vi "HXG2daqFGV.vi"(7 "daqFGV":T2, 8 "error in (no error)":errorcluster) -> (0 "error out":errorcluster, 3 "MAX":T1)   [LabVIEW 2012]
uses:
  HXG2daq.ctl
  Controls/HXG2_MaxConstants.ctl
  <vilib>/DAQmx/write.llb/DAQmx Write (Digital 1D Bool NChan 1Samp 1Line).vi
  <vilib>/DAQmx/write.llb/DAQmx Write (Analog 1D DBL NChan 1Samp).vi
  <resource>/objmgr/daqmx.rc
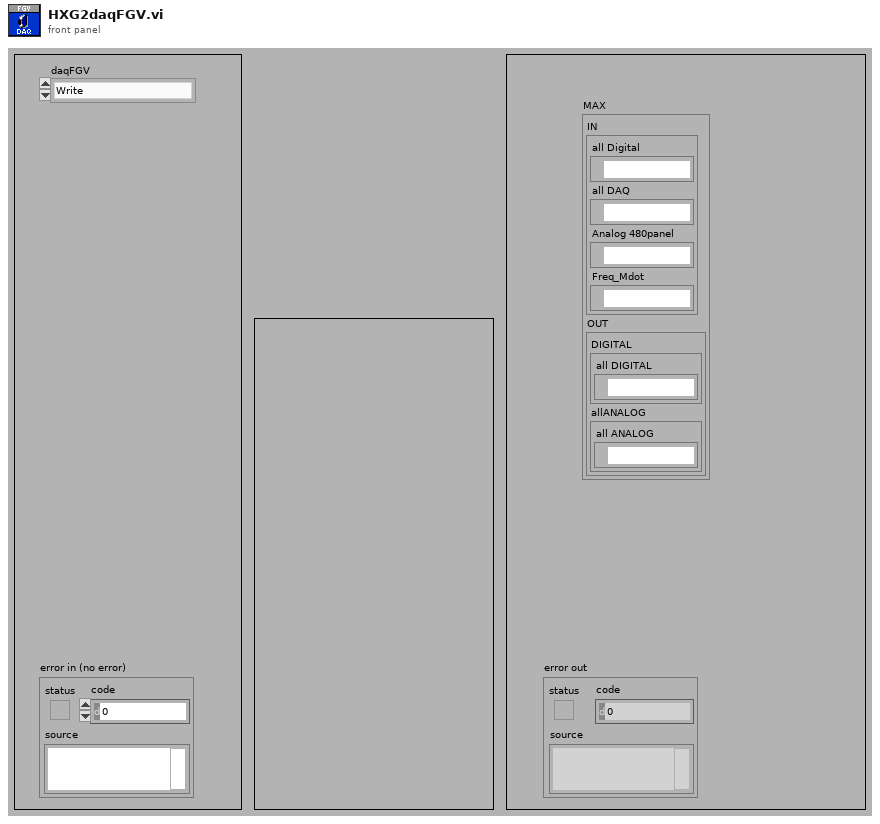
[diagram p1: front panel]
types:
  T1 = typedef "HXG2_MaxConstants.ctl" = cluster{"IN":cluster{"all Digital":refnum<k21>, "all DAQ":refnum<k21>, "Analog 480panel":refnum<k21>, "Freq_Mdot":refnum<k21>}, "OUT":cluster{"DIGITAL":cluster{"all DIGITAL":refnum<k21>}, "allANALOG":cluster{"all ANALOG":refnum<k21>}}}
  T2 = typedef "HXG2daq.ctl" = enum16{"Write", "Pass", "Initialize", "Stop"}
  T3 = cluster{"all Digital":refnum<k21>, "all DAQ":refnum<k21>, "Analog 480panel":refnum<k21>, "Freq_Mdot":refnum<k21>}
  T4 = cluster{"[0]":refnum<k21>, "[1]":refnum<k21>, "[2]":refnum<k21>, "[3]":refnum<k21>}
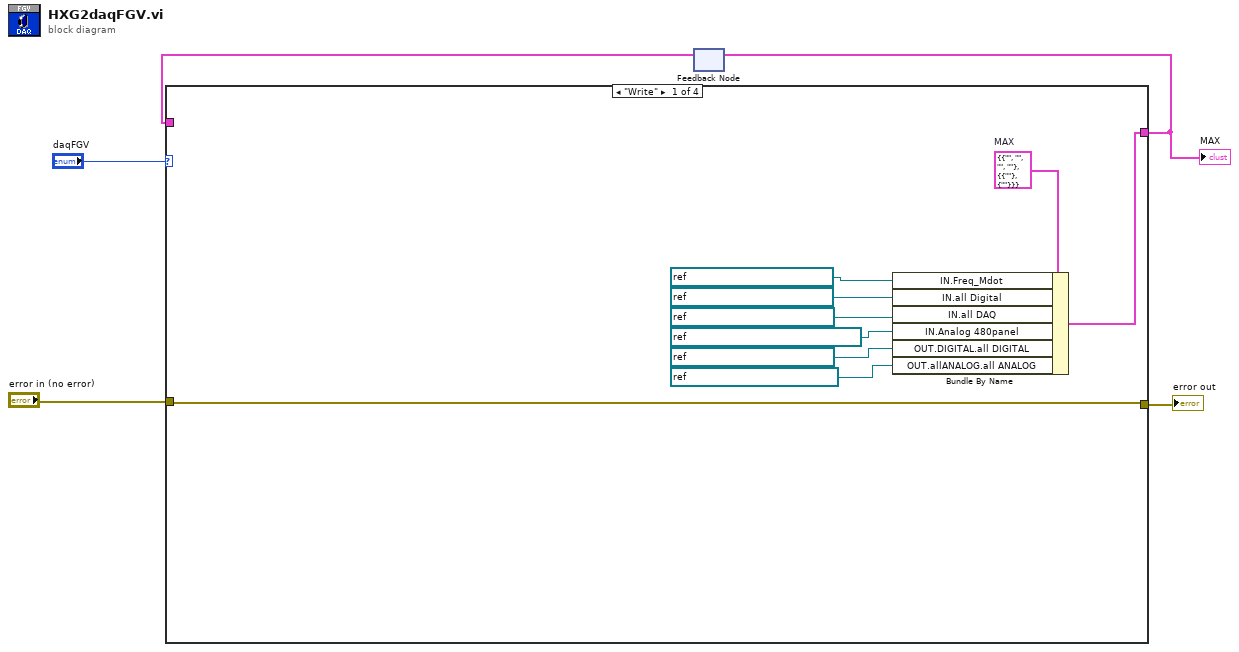
[diagram p0: block diagram]
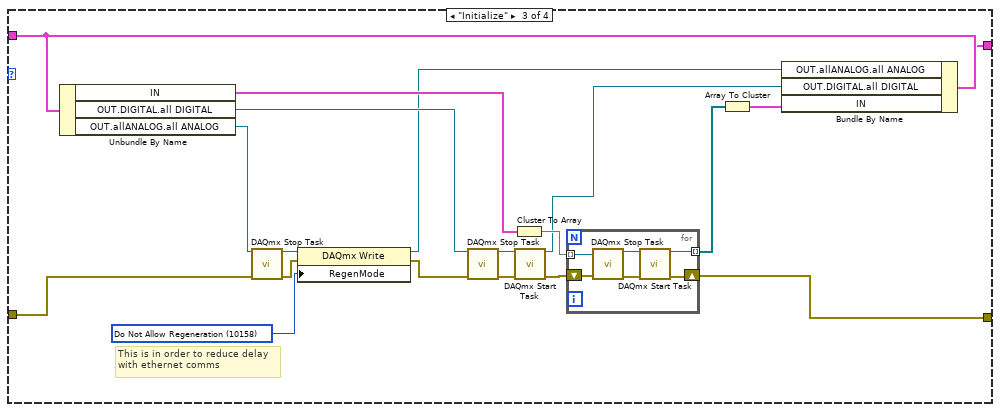
[diagram p3: hidden frame]
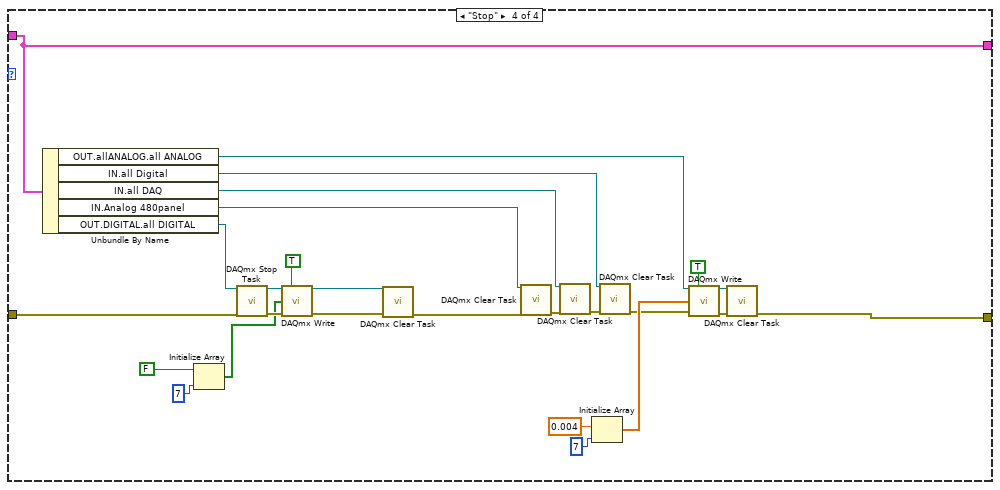
[diagram p4: hidden frame]
diagram:
  n1 = feedback #1() -> (w2:T1)  [unwired: 1 in]
  n2 = case shown="\"Write\"" "daqFGV" {
    tunnel: "error in (no error)" -> [w14 w15 w22 w62]
    tunnel: [w14 w15 w31 w53] -> w4
    tunnel: [w9 w16 w28 w67] -> w3
    tunnel: w2 -> [_ w16 w29 w67]
    frame "Write" {
      w13 = T1 {"IN"={"all Digital"="", "all DAQ"="", "Analog 480panel"="", "Freq_Mdot"=""}, "OUT"={"DIGITAL"={"all DIGITAL"=""}, "allANALOG"={"all ANALOG"=""}}}  # MAX
      n3 = Bundle By Name(cluster=w13, "IN.Freq_Mdot"=refnum<k21> "HX_Cal2_FeqMdot" ("all Digital"), "IN.all Digital"=refnum<k21> "HXCal1_IN_allDIGITAL" ("all Digital"), "IN.all DAQ"=refnum<k21> "HXCal2_IN_ANALOG" ("all DAQ"), "IN.Analog 480panel"=refnum<k21> "HXCal1_IN_ANALOG_480Panel" ("all TC"), "OUT.DIGITAL.all DIGITAL"=refnum<k21> "HXCal1_OUT_allDIGITAL" ("all DIGITAL"), "OUT.allANALOG.all ANALOG"=refnum<k21> "HX_Cal1_OUT_allANALOG" ("all ANALOG")) -> (w9:T1)
    }
    frame "Pass" {
    }
    frame "Initialize" {
      w17 = 10158 items=["Allow Regeneration"=10097, "Do Not Allow Regeneration"=10158] ("RegenMode")
      # "This is in order to reduce delay\nwith ethernet comms"
      n4 = Unbundle By Name(w29) -> ("IN"=w34:T3, "OUT.DIGITAL.all DIGITAL"=w30:refnum<k21>, "OUT.allANALOG.all ANALOG"=w32:refnum<k21>)
      n5 = call <vilib>:"DAQmx Stop Task.vi"("task/channels in"=w32, "error in"=w22) -> ("task out"=w20:refnum<k21>, "error out"=w21:errorcluster)  [unwired: 12 in]
      n6 = property class="DAQmx Write"(reference=w20, error in=w21, "RegenMode"=w17) -> (reference out=w18:refnum<k21>, error out=w19:errorcluster)
      n7 = call <vilib>:"DAQmx Stop Task.vi"("task/channels in"=w30, "error in"=w19) -> ("task out"=w24:refnum<k21>, "error out"=w25:errorcluster)  [unwired: 12 in]
      n8 = Cluster To Array(cluster=w34) -> (array=w33:refnum<k21>[])
      n9 = call <vilib>:"DAQmx Start Task.vi"("task/channels in"=w24, "error in"=w25) -> ("task out"=w23:refnum<k21>, "error out"=w35:errorcluster)  [unwired: 12 in]
      n10 = for {
        shift-right: [w36] -> w31
        shift-left: w35 -> [w41]
        tunnel: w33 -> [w40] mode=indexing
        tunnel: [w37] -> w27 mode=indexing
        n11 = call <vilib>:"DAQmx Stop Task.vi"("task/channels in"=w40, "error in"=w41) -> ("task out"=w39:refnum<k21>, "error out"=w38:errorcluster)  [unwired: 12 in]
        n12 = call <vilib>:"DAQmx Start Task.vi"("task/channels in"=w39, "error in"=w38) -> ("task out"=w37:refnum<k21>, "error out"=w36:errorcluster)  [unwired: 12 in]
      }
      n13 = Array To Cluster(array=w27) -> (cluster=w26:T4)
      n14 = Bundle By Name(cluster=w29, "OUT.allANALOG.all ANALOG"=w18, "OUT.DIGITAL.all DIGITAL"=w23, "IN"=w26) -> (w28:T1)
    }
    frame "Stop" {
      n15 = Unbundle By Name(w67) -> ("OUT.allANALOG.all ANALOG"=w61:refnum<k21>, "IN.all Digital"=w46:refnum<k21>, "IN.all DAQ"=w48:refnum<k21>, "IN.Analog 480panel"=w50:refnum<k21>, "OUT.DIGITAL.all DIGITAL"=w63:refnum<k21>)
      n16 = Initialize Array(FALSE ("auto start"), 7 ("dimension size")) -> (w56:bool[])
      n17 = call <vilib>:"DAQmx Stop Task.vi"("task/channels in"=w63, "error in"=w62) -> ("task out"=w65:refnum<k21>, "error out"=w64:errorcluster)  [unwired: 12 in]
      n18 = call-poly <vilib>:"DAQmx Write.vi"("task/channels in"=w65, "auto start"=TRUE, "data"=w56, "error in"=w64) -> ("task out"=w44:refnum<k21>, "error out"=w43:errorcluster)  [unwired: 9 in, 1 out]
      n19 = call <vilib>:"DAQmx Clear Task.vi"("task in"=w44, "error in"=w43) -> ("error out"=w42:errorcluster)  [unwired: 13 in]
      n20 = call <vilib>:"DAQmx Clear Task.vi"("task in"=w50, "error in"=w42) -> ("error out"=w49:errorcluster)  [unwired: 13 in]
      n21 = call <vilib>:"DAQmx Clear Task.vi"("task in"=w48, "error in"=w49) -> ("error out"=w47:errorcluster)  [unwired: 13 in]
      n22 = Initialize Array(0.004, 7 ("dimension size")) -> (w59:dbl[])
      n23 = call <vilib>:"DAQmx Clear Task.vi"("task in"=w46, "error in"=w47) -> ("error out"=w45:errorcluster)  [unwired: 13 in]
      n24 = call-poly <vilib>:"DAQmx Write.vi"("task/channels in"=w61, "auto start"=TRUE, "data"=w59, "error in"=w45) -> ("task out"=w55:refnum<k21>, "error out"=w54:errorcluster)  [unwired: 9 in, 1 out]
      n25 = call <vilib>:"DAQmx Clear Task.vi"("task in"=w55, "error in"=w54) -> ("error out"=w53:errorcluster)  [unwired: 13 in]
    }
  }
  "error out" <- w4
  "MAX" <- w3
  n26 = feedback-in #1(w3) -> ()
